vi "ProdaNG.Exit.vi"(8 "error in (no error)":errorcluster) -> (0 "error out":errorcluster {"code" format="%.2f"})   [LabVIEW 2016]
doc: "ExitProDll must be called from the Main Thread after all functions have been finished and the program is going to be left. All open connections will be closed and all allocated structures will be released."
uses:
  prodllNG.dll
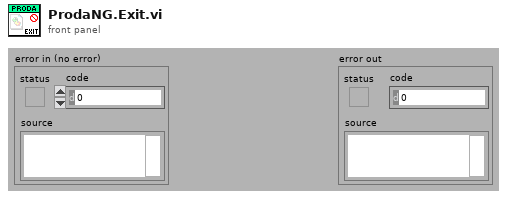
[diagram p1: front panel]
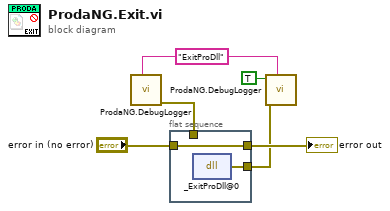
[diagram p0: block diagram]
diagram:
  w3 = "ExitProDll" ("cmd")
  n1 = call "ProdaNG.DebugLogger.vi"("cmd"=w3) -> ("error out"=w1:errorcluster)  [unwired: 10 in]
  n2 = flat-sequence {
    tunnel: "error in (no error)" -> [w8]
    tunnel: [w8] -> w5
    tunnel: [w7] -> w2
    tunnel: w1 -> [_]
    frame #0 {
      n3 = dll-call lib="D:/svn/LineTraceSystem/SOFTWARE/sources/Database/ProdaNG/prodllNG.dll" fn="_ExitProDll@0" ("ProDll.dll:ExitProDll")() -> (error out=w7:errorcluster)  [unwired: 4 in, 1 out]
    }
  }
  n4 = call "ProdaNG.DebugLogger.vi"("cmd"=w3, "error in (no error)"=w2, "done? (F)"=TRUE) -> ()  [unwired: 8 in, 1 out]
  "error out" <- w5
